vi "HandleWin.vi"(8 "error in (no error)":errorcluster, 11 "Pong in":refnum<class "Pong.lvclass">) -> (0 "error out":errorcluster, 3 "Pong out":refnum<class "Pong.lvclass">)   [LabVIEW 2019, in "RT_Game.lvlib" / "Pong.lvclass"]
uses:
  Pong.lvclass
  C:/Users/FreshBob/Dropbox/VIs/myRIO_GameConsole/RT/RT_Game/Game/Game.lvclass
  Winners.ctl
  Pong.lvclass/Pong.ctl
  Game/Coordinate.ctl
  PongBall/PongBall.lvclass
  C:/Users/FreshBob/Dropbox/VIs/myRIO_GameConsole/RT/RT_Game/RT_Sprite/RT_Sprite.lvclass
  Game/Game.lvclass/Game.ctl
  Game/Read Sprite3.vi
  Game/Write Sprite3.vi
  RT_Sprite/RT_Sprite.lvclass
  Game/Game.lvclass
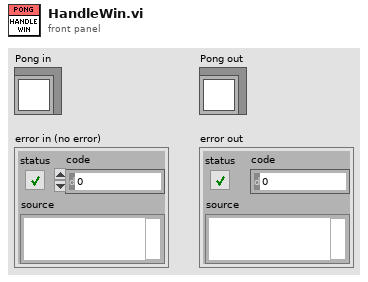
[diagram p1: front panel]
types:
  T1 = typedef "RT_Game.lvlib/Pong.lvclass/Winners.ctl" = enum16{"None", "Player1", "Player2"}
  T2 = typedef "RT_Game.lvlib/Game.lvclass/Coordinate.ctl" = cluster{"x":dbl, "y":dbl}
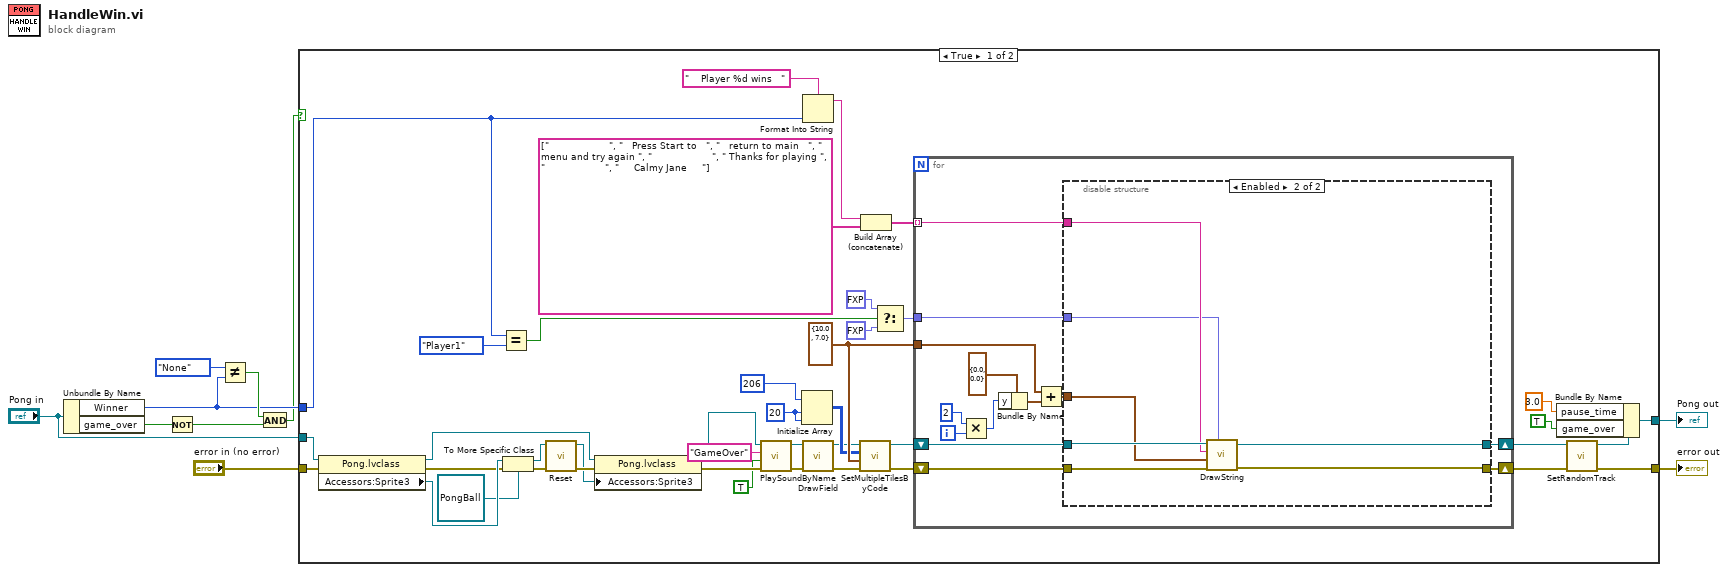
[diagram p0: block diagram]
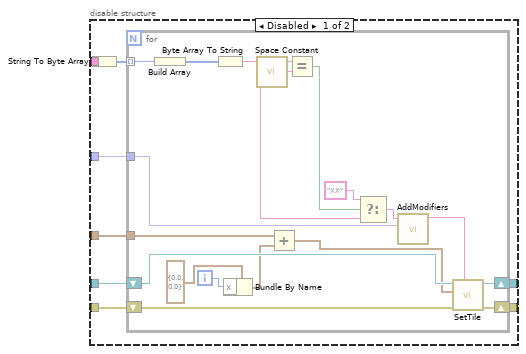
[diagram p2: hidden frame]
diagram:
  n1 = Unbundle By Name("Pong in") -> ("Winner"=w5:T1, "game_over"=w6:bool)
  n2 = Not(x=w6) -> (.not. x?=w4:bool)
  n3 = Not Equal?(x=Winners."None", y=w5) -> (x != y?=w7:bool)
  n4 = And(x=w7, y=w4) -> (x .and. y?=w3:bool)
  n5 = case shown="True" w3 {
    tunnel: [w16 w98] -> w10
    tunnel: [w32 w99] -> w9
    tunnel: w5 -> [w38 _]
    tunnel: "Pong in" -> [w24 w99]
    tunnel: "error in (no error)" -> [w23 w98]
    frame True {
      w40 = 20 ("dimension size")
      w41 = T2 {"x"=10.0, "y"=7.0} ("Coordinate")
      n6 = property class="Pong.lvclass"(reference=w24, error in=w23) -> (reference out=w20:refnum<class "Pong.lvclass">, error out=w26:errorcluster, "Accessors:Sprite3"=w27:refnum<class "RT_Sprite.lvclass">)
      n7 = Equal?(x=w38, y=Winners."Player1") -> (x = y?=w35:bool)
      n8 = To More Specific Class(target class=refnum<class "PongBall.lvclass"> refnum ("RT_Game.lvlib:PongBall.lvclass"), reference=w27, error in=w26) -> (specific class reference=w22:refnum<class "PongBall.lvclass">, error out=w21:errorcluster)
      n9 = call "Reset.vi"("error in (no error)"=w21, "PongBall in"=w22) -> ("error out"=w49:errorcluster, "PongBall out"=w17:refnum<class "PongBall.lvclass">)  [unwired: 8 in]
      n10 = property class="Pong.lvclass"(reference=w20, error in=w49, "Accessors:Sprite3"=w17) -> (reference out=w18:refnum<class "Pong.lvclass">, error out=w19:errorcluster)
      n11 = call "PlaySoundByName.vi"("error in (no error)"=w19, "Overwrite"=TRUE, "Name"="GameOver", "Game in"=w18) -> ("error out"=w29:errorcluster, "Game out"=w28:refnum<class "Pong.lvclass">)  [unwired: 6 in]
      n12 = Initialize Array(u32 206 ("dimension size"), w40, w40) -> (w39:u32[][])
      n13 = Format Into String(format string="    Player %d wins   " ("String"), w38) -> (resulting string=w44:string)  [unwired: 2 in, 1 out]
      n14 = call "DrawField.vi"("error in (no error)"=w29, "Pong in"=w28) -> ("error out"=w31:errorcluster, "Pong out"=w30:refnum<class "Pong.lvclass">)  [unwired: 8 in]
      n15 = call "SetMultipleTilesByCode.vi"("error in (no error)"=w31, "Position"=w41, "TileCodes"=w39, "Game in"=w30) -> ("error out"=w43:errorcluster, "Game out"=w42:refnum<class "Pong.lvclass">)  [unwired: 6 in]
      n16 = Build Array (concatenate)(w44, string[] ["                    ", "   Press Start to   ", "   return to main   ", " menu and try again ", "                    ", " Thanks for playing ", "                    ", "     Calmy Jane     "] ("String")) -> (w45:string[])
      n17 = Select(t=fxp<+,3,3> 1.0, s=w35, f=fxp<+,3,3> 2.0 ("Color (7=white)")) -> (s? t:f=w33:fxp<+,3,3>)
      n18 = for {
        tunnel: w45 -> [w60] mode=indexing
        shift-right: [w61] -> w51
        shift-left: w43 -> [w64]
        shift-right: [w62] -> w15
        shift-left: w42 -> [w63]
        tunnel: w41 -> [w59]
        tunnel: w33 -> [w52]
        i -> [w55]
        n19 = Multiply(x=2, y=w55) -> (x*y=w54:i32)
        n20 = Bundle By Name(cluster=T2 {"x"=0.0, "y"=0.0} ("x"), "y"=w54) -> (w56:T2)
        n21 = Add(x=w59, y=w56) -> (x+y=w58:T2)
        n22 = disable-structure shown="Enabled" {
          disable-tunnel: w64 -> [w72 w96]
          disable-tunnel: w63 -> [w71 w97]
          disable-tunnel: [w70 w94] -> w62
          disable-tunnel: [w69 w95] -> w61
          disable-tunnel: w60 -> [w68 w93]
          disable-tunnel: w58 -> [w67 w92]
          disable-tunnel: w52 -> [w65 w91]
          frame Disabled {
            n23 = String To Byte Array(string=w68) -> (unsigned byte array=w66:u8[])
            n24 = for {
              shift-right: [w89] -> w69
              shift-left: w72 -> [w90]
              shift-right: [w87] -> w70
              shift-left: w71 -> [w88]
              tunnel: w66 -> [w86] mode=indexing
              tunnel: w67 -> [w84]
              tunnel: w65 -> [w73]
              i -> [w80]
              n25 = Build Array(w86) -> (w85:u8[])
              n26 = Byte Array To String(unsigned byte array=w85) -> (string=w76:string)
              n27 = Bundle By Name(cluster=T2 {"x"=0.0, "y"=0.0} ("y"), "x"=w80) -> (w81:T2)
              n28 = call <vilib>:"Space Constant.vi"() -> ("String"=w78:string)
              n29 = Add(x=w84, y=w81) -> (x+y=w83:T2)
              n30 = Equal?(x=w76, y=w78) -> (x = y?=w75:bool)
              n31 = Select(t="XX", s=w75, f=w76) -> (s? t:f=w77:string)
              n32 = call "AddModifiers.vi"("ReplaceColor (1=red)"=w73, "String in"=w77) -> ("String out"=w79:string)  [unwired: 9 in]
              n33 = call "SetTile.vi"("TileCode"=w79, "error in (no error)"=w90, "Coordinates"=w83, "Game in"=w88) -> ("error out"=w89:errorcluster, "Game out"=w87:refnum<class "Pong.lvclass">)  [unwired: 6 in]
            }
          }
          frame Enabled {
            n34 = call "DrawString.vi"("Color (7=white)"=w91, "error in (no error)"=w96, "Coordinate"=w92, "String"=w93, "RT_Game.lvlib:Game.lvclass"=w97) -> ("error out"=w95:errorcluster, "RT_Game.lvlib:Game.lvclass 2"=w94:refnum<class "Pong.lvclass">)  [unwired: 5 in]
          }
        }
      }
      n35 = call "SetRandomTrack.vi"("error in (no error)"=w51, "Game in"=w15) -> ("error out"=w16:errorcluster, "Game out"=w14:refnum<class "Pong.lvclass">)  [unwired: 8 in]
      n36 = Bundle By Name(cluster=w14, "pause_time"=3.0, "game_over"=TRUE) -> (w32:refnum<class "Pong.lvclass">)
    }
    frame False {
    }
  }
  "error out" <- w10
  "Pong out" <- w9
